vi "convert tif to jpg.vi"() -> ()   [LabVIEW 2014]
uses:
  <vilib>/Utility/file.llb/Write To Spreadsheet File (DBL).vi
panel:
  out "Image":T1(plugin-control)
  in  "Correlation Time (s)":dbl
  in  "Max Voltage":dbl
  in  "Min Voltage":dbl
  in  "Frames":i32
  in  "Sigma":dbl
  in  "Offset Voltage":dbl
  out "Save Directory":path
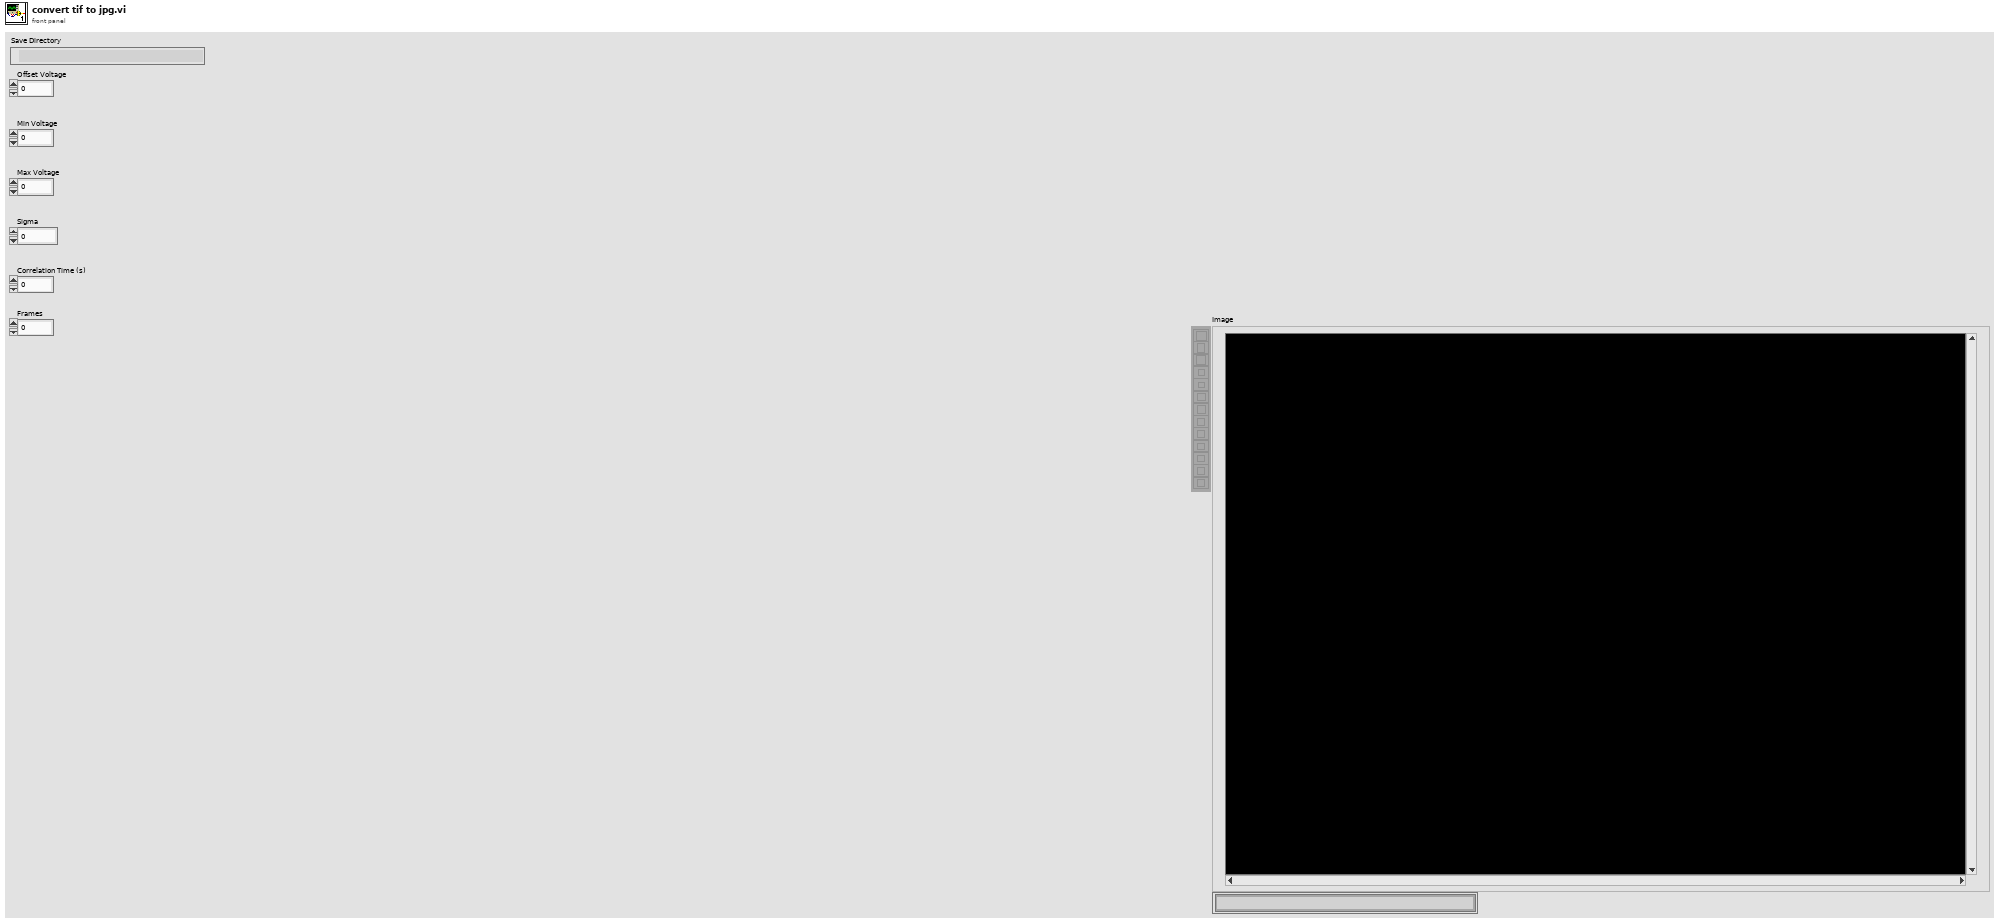
[diagram p1: front panel]
types:
  T1 = typedef "IMAQ Image.ctl" = refnum<image>
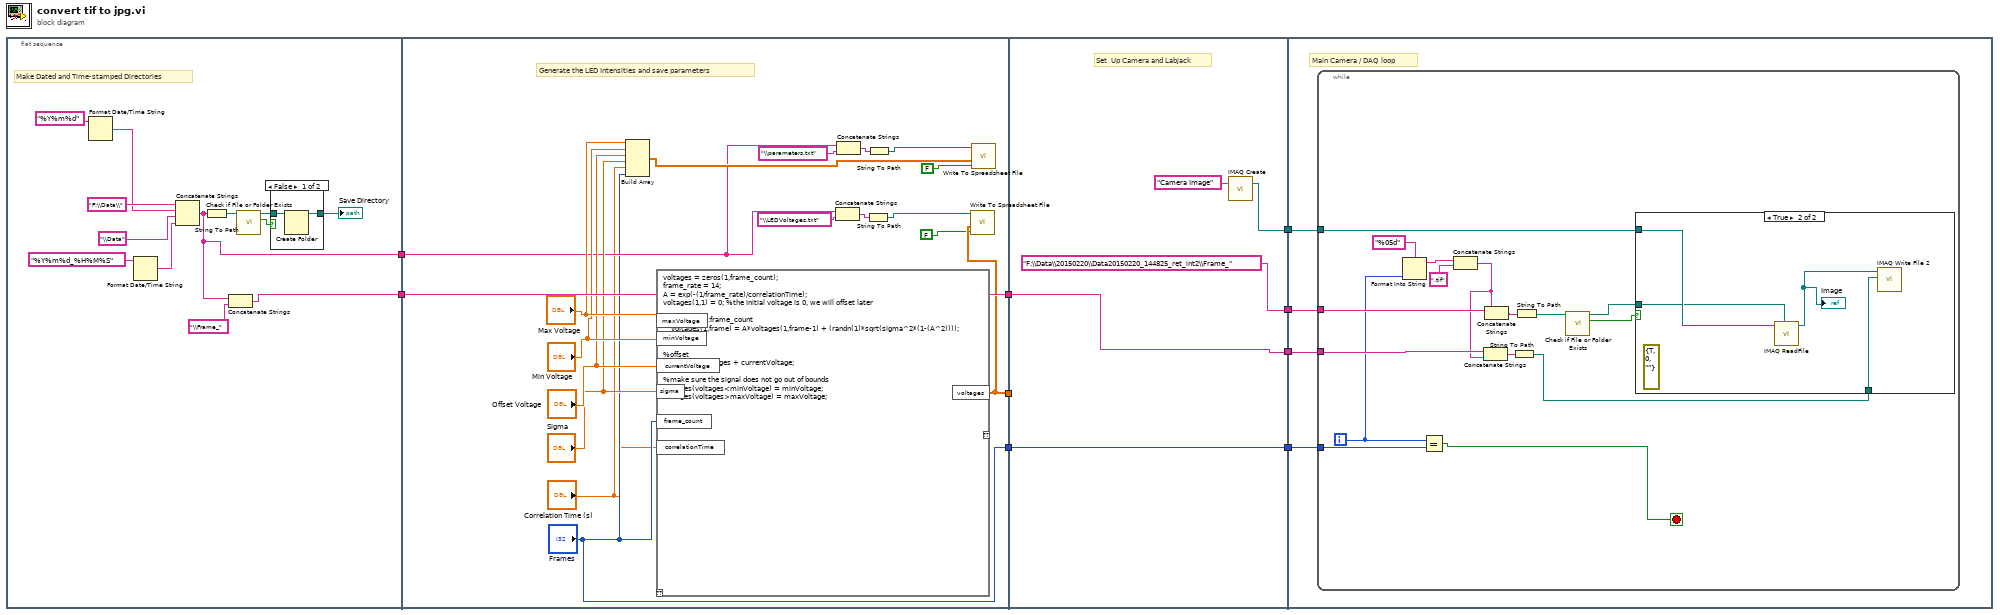
[diagram p0: block diagram]
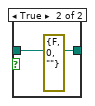
[diagram p2: hidden frame]
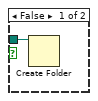
[diagram p3: hidden frame]
diagram:
  n1 = flat-sequence {
    tunnel: [w12] -> w4
    tunnel: [w10] -> w3
    tunnel: [w41] -> w8
    tunnel: [w39] -> w7
    tunnel: ["Frames"] -> w6
    tunnel: w3 -> [w28]
    tunnel: w4 -> [w41]
    tunnel: w8 -> [w45]
    tunnel: ["F:\\Data\\20150220\\Data20150220_144825_ret_int2\\Frame_"] -> w9
    tunnel: w7 -> [_]
    tunnel: w6 -> [w48]
    tunnel: [w48] -> w5
    tunnel: [w45] -> w2
    tunnel: [w46] -> w1
    tunnel: w2 -> [w50]
    tunnel: w5 -> [w51]
    tunnel: w9 -> [w52]
    tunnel: w1 -> [w49]
    frame #0 {
      # "Make Dated and Time-stamped Directories"
      n2 = Format Date/Time String(time format string (%c)="%Y%m%d") -> (date/time string=w13:string)  [unwired: 2 in]
      n3 = Format Date/Time String(time format string (%c)="%Y%m%d_%H%M%S") -> (date/time string=w17:string)  [unwired: 2 in]
      n4 = Concatenate Strings("F:\\Data\\", w13, "\\Data", w17) -> (w10:string)
      n5 = String To Path(string=w10) -> (path=w16:path)
      n6 = Concatenate Strings(w10, "\\Frame_") -> (w12:string)
      n7 = call <vilib>:"Check if File or Folder Exists.vi"("path"=w16) -> ("file or folder exists?"=w21:bool, "dup path"=w20:path)  [unwired: 8 in, 1 out]
      n8 = case shown="False" w21 {
        tunnel: [w23 w25] -> w15
        tunnel: w20 -> [w24 w25]
        frame False {
          n9 = Create Folder(path (use dialog)=w24) -> (created path=w23:path)  [unwired: 2 in, 2 out]
        }
        frame True {
          (unwired) errorcluster {"status"=FALSE, "code"=0, "source"=""} ("error out")
        }
      }
      "Save Directory" <- w15
    }
    frame #1 {
      # "Generate the LED Intensities and save parameters"
      n10 = Build Array("Max Voltage", "Min Voltage", "Offset Voltage", "Sigma", "Correlation Time (s)", "Frames") -> (w29:dbl[])
      n11 = script code="voltages = zeros(1,frame_count);\nframe_rate = 14;\nA = exp(-(1/frame_rate)/correlationTime);\nvoltages(1,1) = 0; %the initial voltage is 0, we will offset later\n\nfor frame = 2:frame_count\n    voltages(1,frame) = A*voltages(1,frame-1) + (randn(1)*sqrt(sigma^2*(1-(A^2))));\nend\n\n%offset\nvoltages = voltages + currentVoltage;\n\n%make sure the signal does not go out of bounds\nvoltages(voltages<minVoltage) = minVoltage;\nvoltages(voltages>maxVoltage) = maxVoltage;"("currentVoltage"="Offset Voltage", "frame_count"="Frames", "sigma"="Sigma", "minVoltage"="Min Voltage", "maxVoltage"="Max Voltage", "correlationTime"="Correlation Time (s)") -> ("voltages"=w39:dbl[])  [unwired: 1 in, 1 out]
      n12 = Concatenate Strings(w28, "\\LEDVoltages.txt") -> (w43:string)
      n13 = Concatenate Strings(w28, "\\parameters.txt") -> (w33:string)
      n14 = String To Path(string=w43) -> (path=w42:path)
      n15 = String To Path(string=w33) -> (path=w32:path)
      n16 = call-poly <vilib>:"Write To Spreadsheet File.vi"("append to file? (new file:F)"=FALSE, "1D data"=w39, "file path (dialog if empty)"=w42) -> ()  [unwired: 5 in, 1 out]
      n17 = call-poly <vilib>:"Write To Spreadsheet File.vi"("append to file? (new file:F)"=FALSE, "1D data"=w29, "file path (dialog if empty)"=w32) -> ()  [unwired: 5 in, 1 out]
    }
    frame #2 {
      # "Set  Up Camera and Labjack"
      n18 = call "IMAQ Create"("Image Name"="Camera Image") -> ("New Image"=w46:T1)  [unwired: 4 in, 1 out]
    }
    frame #3 {
      # "Main Camera / DAQ loop"
      n19 = while {
        tunnel: w52 -> [w63]
        tunnel: w51 -> [w65]
        tunnel: w50 -> [w61]
        tunnel: w49 -> [w54]
        i -> [w58]
        stop <- w64 stop-if-true
        n20 = Format Into String(format string="%05d" ("string"), w58) -> (resulting string=w67:string)  [unwired: 2 in, 1 out]
        n21 = Equal?(x=w58, y=w65) -> (x = y?=w64:bool)
        n22 = Concatenate Strings(w67, ".tif" ("string")) -> (w60:string)
        n23 = Concatenate Strings(w61, w60) -> (w59:string)
        n24 = Concatenate Strings(w63, w60) -> (w62:string)
        n25 = String To Path(string=w59) -> (path=w53:path)
        n26 = String To Path(string=w62) -> (path=w55:path)
        n27 = call <vilib>:"Check if File or Folder Exists.vi"("path"=w55) -> ("file or folder exists?"=w57:bool, "dup path"=w56:path)  [unwired: 8 in, 1 out]
        n28 = case shown="True" w57 {
          tunnel: w56 -> [w69 w71]
          tunnel: w54 -> [_ w73]
          tunnel: w53 -> [_ w72]
          frame False {
            n29 = Create Folder(path (use dialog)=w69) -> ()  [unwired: 2 in, 3 out]
          }
          frame True {
            (unwired) errorcluster {"status"=TRUE, "code"=0, "source"=""} ("error out")
            n30 = call "IMAQ ReadFile"("File Path"=w71, "Image"=w73) -> ("Image Out"=w70:T1)  [unwired: 5 in, 4 out]
            "Image" <- w70
            n31 = call-poly "IMAQ Write File 2"("File Path"=w72, "Image"=w70) -> ()  [unwired: 8 in, 2 out]
          }
        }
      }
    }
  }
